vi "Среднее по ROI.vi"() -> ()   [LabVIEW 2018]
uses:
  <vilib>/Analysis/NI_AALBase.lvlib
panel:
  in  "Стоп":bool
  out "Image":T1(plugin-control)
  out "СЗ, ед":u16
  out "СКО, ед.":u16
  in  "Анализ":path=path "C:/Users/agest/Downloads/MT9V024IA7XTM/MT9V024IA7XTM/FRAMES/Первый кадр.PNG"
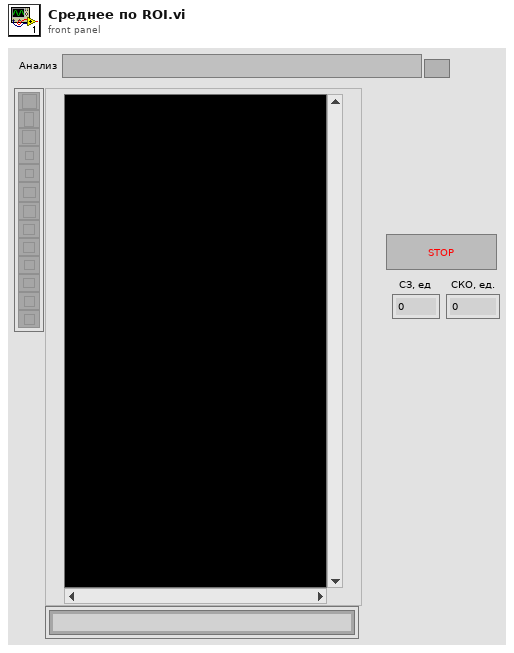
[diagram p1: front panel]
types:
  T1 = typedef "IMAQ Image.ctl" = refnum<image>
  T2 = typedef "Image Type" = u32
  T3 = cluster{"Global Rectangle":i32[], "Contours":cluster{"Contour Type":u32, "ROI Type":u32, "Points":i32[]}[]}
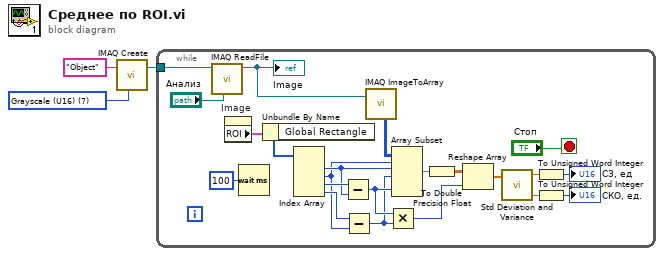
[diagram p0: block diagram]
diagram:
  w2 = T2 7 items=["Grayscale (U8)", "Grayscale (I16)", "Grayscale (SGL)", "Complex (CSG)", "RGB (U32)", "HSL (U32)", "RGB (U64)", "Grayscale (U16)"] ("Image Type")
  n1 = call "IMAQ Create"("Image Name"="Object", "Image Type"=w2) -> ("New Image"=w3:T1)  [unwired: 3 in, 1 out]
  n2 = while {
    tunnel: w3 -> [w6]
    stop <- "Стоп" stop-if-true
    n3 = call "IMAQ ReadFile"("File Path"="Анализ", "Image"=w6) -> ("Image Out"=w8:T1)  [unwired: 5 in, 4 out]
    "Image" <- w8
    n4 = property on="Image" class="ImageControl"() -> ("ROI"=w10:T3)  [unwired: 2 in, 2 out]
    n5 = Wait (ms)(milliseconds to wait=u32 100) -> ()  [unwired: 1 out]
    n6 = Unbundle By Name(w10) -> ("Global Rectangle"=w18:i32[])
    n7 = Index Array(array=w18) -> (element #1=w16:i32, element #2=w13:i32, element #3=w17:i32, element #4=w14:i32)  [unwired: 4 in]
    n8 = Subtract(x=w17, y=w16) -> (x-y=w15:i32)
    n9 = Subtract(x=w14, y=w13) -> (x-y=w12:i32)
    n10 = call "IMAQ ImageToArray"("Image"=w8) -> ("Image Pixels (U16)"=w7:u16[][])  [unwired: 3 in, 4 out]
    n11 = Multiply(x=w15, y=w12) -> (x*y=w25:i32)
    n12 = Array Subset(array=w7, index (row)=w13, length (row)=w12, index (col)=w16, length (col)=w15) -> (w11:u16[][])
    n13 = To Double Precision Float(number=w11) -> (double precision float=w22:dbl[][])
    n14 = Reshape Array(w22, w25) -> (w21:dbl[])
    n15 = call <vilib>:"Std Deviation and Variance.vi"("X"=w21) -> ("mean"=w23:dbl, "standard deviation"=w20:dbl)  [unwired: 1 in, 1 out]
    n16 = To Unsigned Word Integer(number=w23) -> (unsigned 16bit integer=→"СЗ, ед":u16)
    n17 = To Unsigned Word Integer(number=w20) -> (unsigned 16bit integer=→"СКО, ед.":u16)
  }
